vi "GA_Main.vi"() -> ()   [LabVIEW 2018]
uses:
  Control/GA_parameter.ctl
  GA_Global.vi
panel:
  out "Waveform Chart":dbl(graph)=549.9986119849859
  out "subarray":i32[](array[numeric])=[14, 4, 7, 10, 17, 12, 16, 8, 1, 5, 11, 9, 6, 19, 18, 2, 3, 0, 15, 13]
  out "Total Distance":string="549.999"
  out "LOOP":i32=27
  out "XY Graph":cluster{dbl[], dbl[]}[](graph)=[{[0.031661203846429675, 0.5532222561949678, 0.30691650564629724, 0.06216977035211335, 0.815313965925324, 0.7144476383368001, 0.9183677482928667, 0.7779446521382751, 0.4795905054607119, 0.8720375774801024, 0.6403926058667326, 0.7032068224156323, 0.9264410023695555, 0.9102101763051438, 0.3326121413993002, 0.5285409666086607, 0.7491286526018293, 0.8128137275182715, 0.3049377272998468, 0.7442087892303242], [0.6842538606641266, 0.9715325523992502, 0.07947091564951703, 0.3503212954831587, 0.7099335261736506, 0.16504071857534863, 0.19032954174069538, 0.4737202343719036, 0.7220071904670999, 0.1514388717286499, 0.7696046404381676, 0.13186927970936702, 0.6676306082167485, 0.11509432730944802, 0.6153810691316783, 0.6948516575854419, 0.5005740424024072, 0.8454498427949864, 0.03208490125358865, 0.06140943350154693]}, {[0.815313965925324, 0.7779446521382751, 0.6403926058667326, 0.8128137275182715, 0.9264410023695555, 0.7491286526018293, 0.7144476383368001, 0.7032068224156323, 0.8720375774801024, 0.7442087892303242, 0.3049377272998468, 0.30691650564629724, 0.9102101763051438, 0.9183677482928667, 0.3326121413993002, 0.06216977035211335, 0.031661203846429675, 0.4795905054607119, 0.5532222561949678, 0.5285409666086607], [0.7099335261736506, 0.4737202343719036, 0.7696046404381676, 0.8454498427949864, 0.6676306082167485, 0.5005740424024072, 0.16504071857534863, 0.13186927970936702, 0.1514388717286499, 0.06140943350154693, 0.03208490125358865, 0.07947091564951703, 0.11509432730944802, 0.19032954174069538, 0.6153810691316783, 0.3503212954831587, 0.6842538606641266, 0.7220071904670999, 0.9715325523992502, 0.6948516575854419]}]
  in  "Stop Button":bool
  in  "Parameter":T1={"N_CITIES"=20, "POP_SIZE"=800, "N_GENERATIONS"=1200, "CROSS_RATE"=0.1, "MUTATE_RATE"=0.02}
  out "Title":string="LabVIEW and Genetic Algorithm-Travel Sales Problem-V2"
  # "Ricky"
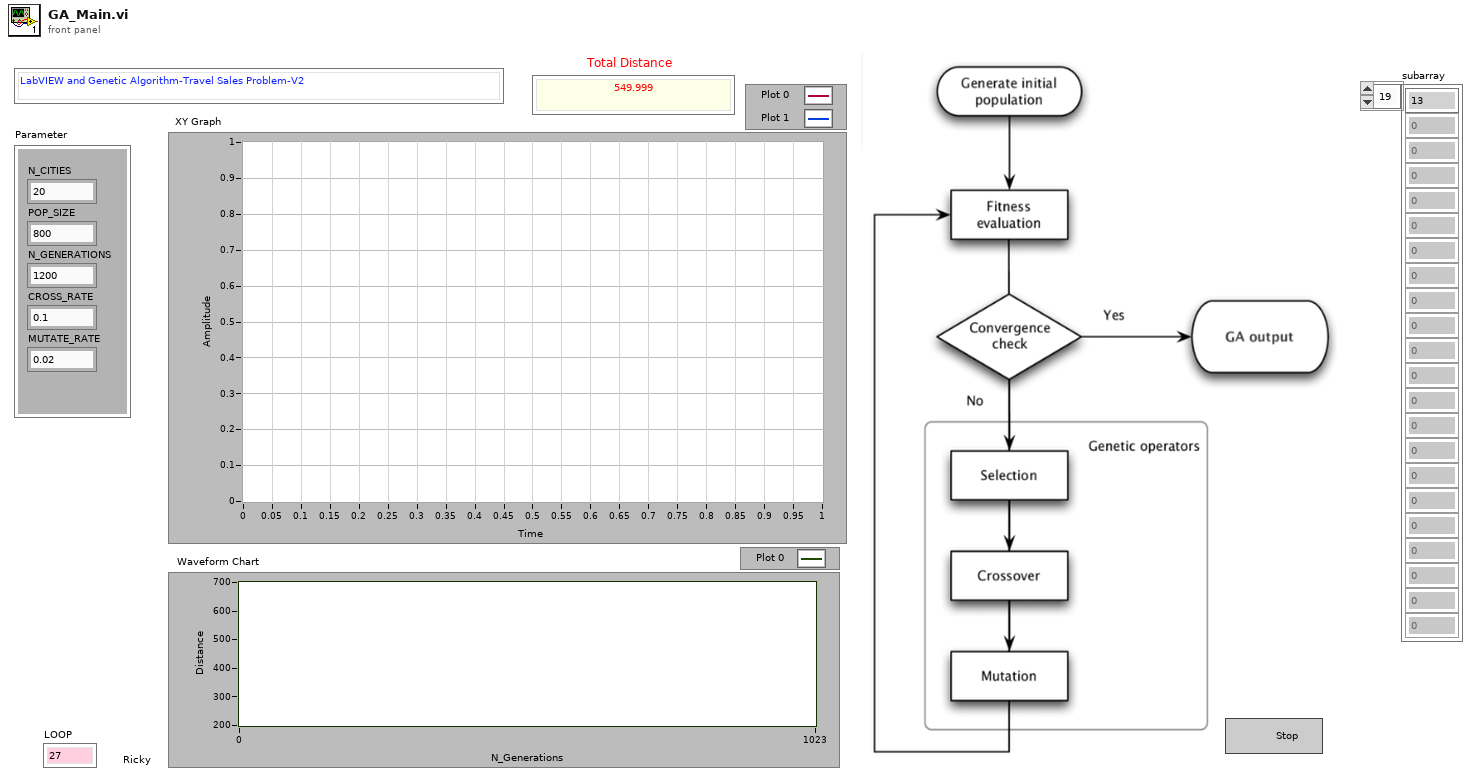
[diagram p1: front panel]
types:
  T1 = typedef "GA_parameter.ctl" = cluster{"N_CITIES":i32, "POP_SIZE":i32, "N_GENERATIONS":i32, "CROSS_RATE":dbl, "MUTATE_RATE":dbl}
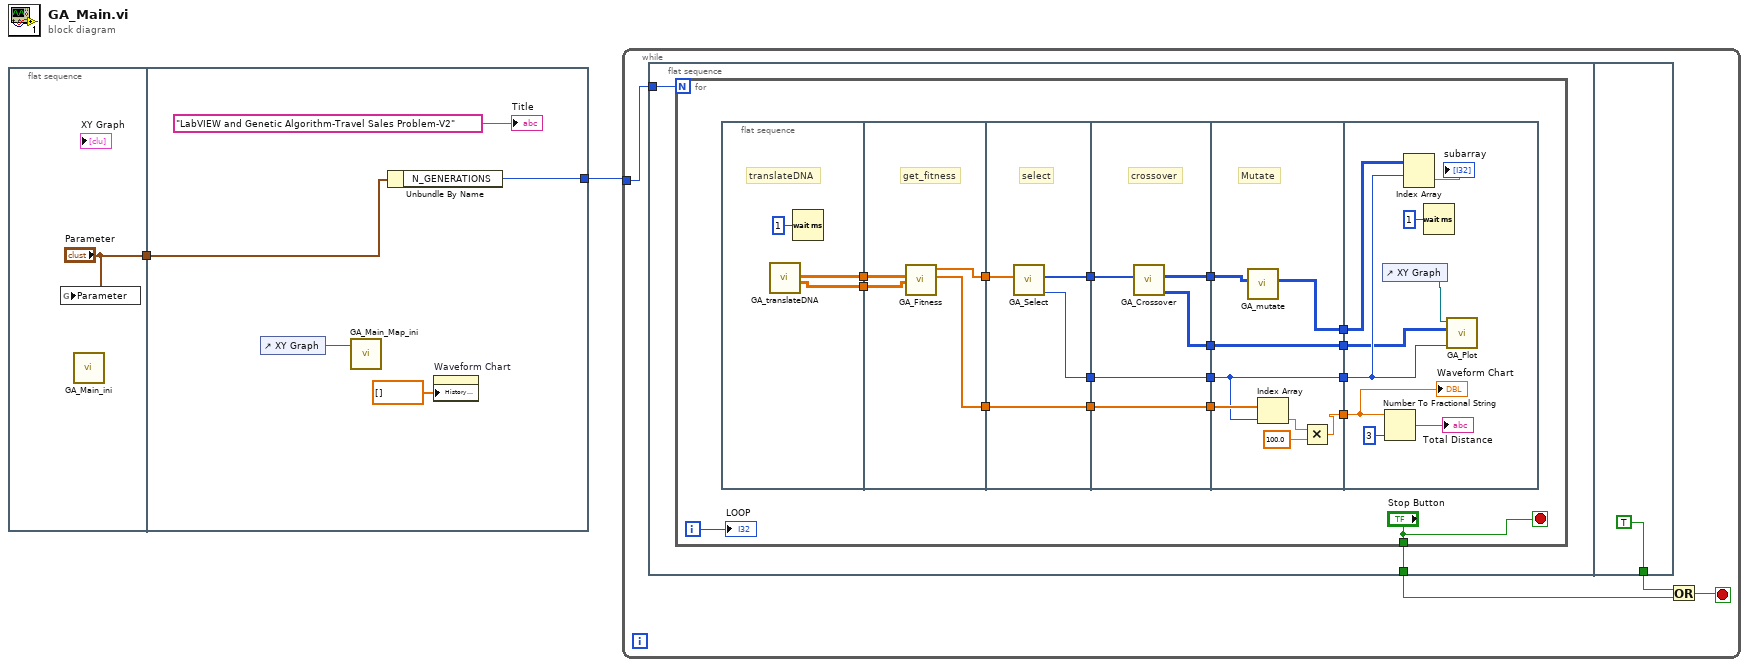
[diagram p0: block diagram]
diagram:
  n1 = flat-sequence {
    tunnel: ["Parameter"] -> w2
    tunnel: w2 -> [w6]
    tunnel: [w5] -> w1
    frame #0 {
      n2 = global write "GA_Global.vi" "Parameter"("Parameter") -> ()
      n3 = call "GA_Main_ini.vi"() -> ()  [unwired: 12 in]
    }
    frame #1 {
      n4 = control-ref of="XY Graph"() -> (w8:refnum<vi>)
      n5 = call "GA_Main_Map_ini.vi"("reference"=w8) -> ()  [unwired: 11 in]
      n6 = Unbundle By Name(w6) -> ("N_GENERATIONS"=w5:i32)
      n7 = property on="Waveform Chart" class="WFChart (strict)"("History Data"=dbl[] []) -> ()  [unwired: 2 in, 2 out]
      "Title" <- "LabVIEW and Genetic Algorithm-Travel Sales Problem-V2" ("Title")
    }
  }
  n8 = while {
    tunnel: w1 -> [w12]
    stop <- w11 stop-if-true
    n9 = flat-sequence {
      tunnel: w12 -> [w14]
      tunnel: [w13] -> w9
      tunnel: [TRUE] -> w10
      frame #0 {
        n10 = for {
          N: w14 -> [_]
          tunnel: ["Stop Button"] -> w13
          i -> [w23]
          stop <- "Stop Button" stop-if-true
          n11 = flat-sequence {
            tunnel: [w34] -> w31
            tunnel: [w33] -> w30
            tunnel: w31 -> [w38]
            tunnel: w30 -> [w37]
            tunnel: [w35] -> w29
            tunnel: [w36] -> w22
            tunnel: w29 -> [w42]
            tunnel: [w41] -> w28
            tunnel: [w40] -> w24
            tunnel: w22 -> [w39]
            tunnel: [w39] -> w20
            tunnel: w28 -> [w47]
            tunnel: [w46] -> w27
            tunnel: [w45] -> w25
            tunnel: w24 -> [w45]
            tunnel: [w44] -> w21
            tunnel: w20 -> [w44]
            tunnel: [w43] -> w15
            tunnel: w27 -> [w51]
            tunnel: [w48] -> w26
            tunnel: w25 -> [w48]
            tunnel: w21 -> [w55]
            tunnel: [w52] -> w19
            tunnel: [w50] -> w18
            tunnel: [w49] -> w16
            tunnel: w15 -> [w49]
            tunnel: w26 -> [w59]
            tunnel: w19 -> [w57]
            tunnel: w18 -> [w60]
            tunnel: w16 -> [w56]
            frame #0 {
              # "translateDNA"
              n12 = call "GA_translateDNA.vi"() -> ("line_y (500, 20)"=w33:dbl[][], "line_x (500, 20)"=w34:dbl[][])  [unwired: 10 in]
              n13 = Wait (ms)(milliseconds to wait=u32 1) -> ()  [unwired: 1 out]
            }
            frame #1 {
              # "get_fitness"
              n14 = call "GA_Fitness.vi"("line_y (500, 20)"=w37, "line_x (500, 20)"=w38) -> ("total_distance(500)"=w36:dbl[], "fitness(500)"=w35:dbl[])  [unwired: 6 in, 1 out]
            }
            frame #2 {
              # "select"
              n15 = call "GA_Select.vi"("fitness(500)_1"=w42) -> ("max index(es)"=w40:i32, "pop[idx]_500"=w41:i32[])  [unwired: 9 in]
            }
            frame #3 {
              # "crossover"
              n16 = call "GA_Crossover.vi"("pop[idx]_500"=w47) -> ("pop(500*20) 2"=w43:i32[][], "pop(500*20)"=w46:i32[][])  [unwired: 9 in]
            }
            frame #4 {
              # "Mutate"
              n17 = call "GA_mutate.vi"("pop(500*20)"=w51) -> ("pop(500*20) 2"=w50:i32[][])  [unwired: 10 in]
              n18 = Index Array(array=w55, index=w48) -> (element=w54:dbl)
              n19 = Multiply(x=w54, y=100.0) -> (x*y=w52:dbl)
            }
            frame #5 {
              n20 = control-ref of="XY Graph"() -> (w64:refnum<vi>)
              n21 = Number To Fractional String(number=w57, precision (6)=i16 3) -> (F-format string=→"Total Distance":string)  [unwired: 2 in]
              n22 = Index Array(array=w60, index (row)=w59) -> (element=→"subarray":i32[])  [unwired: 1 in]
              n23 = Wait (ms)(milliseconds to wait=u32 1) -> ()  [unwired: 1 out]
              n24 = call "GA_Plot.vi"("max index(es)"=w59, "pop(500*20)"=w56, "reference"=w64) -> ()  [unwired: 9 in]
              "Waveform Chart" <- w57
            }
          }
          "LOOP" <- w23
        }
      }
      frame #1 {
      }
    }
    n25 = Or(x=w10, y=w9) -> (x .or. y?=w11:bool)
  }
